vi "hdf5 image save.vi"(6 "class path":path, 7 "Save Image Path":path, 8 "error in (no error)":errorcluster, 9 "Status":T3, 10 "image #":i16=1, 11 "Refnum in":T2) -> (0 "error out":errorcluster)   [LabVIEW 2020, in "Point Grey Camera.lvclass"]
uses:
  Point Grey Camera.lvclass
  1st or last shot of scan.ctl
  <vilib>/vision/Image Controls.llb/IMAQ Image.ctl
panel:
  out "scan number":string
  in  "Python version":string="3.8"
  out "module path":path=path "C:/GEECS/Developers Version/source/Axel/openPMD-CCD/openpmd_ccd_labview.py"
  out "camera name":string
  out "Image Type 2":T1 items=["Grayscale (U8)", "Grayscale (I16)", "Grayscale (SGL)", "Complex (CSG)", "RGB (U32)", "HSL (U32)", "RGB (U64)", "Grayscale (U16)"]
  # "Error 1671 occurred at Python Node in Point Grey Camera.lvclass:hdf5 image save.vi->Point Grey Camera.lvclass:imaq save GEECS.vi->Point Grey Camera.lvclass:Save.vi->Device_control.vi\n\nPossible reason(s):\n\nLabVIEW: (Hex 0x687) There was an error in executing the specified function.\n\n\nModule Path: C:\\GEECS\\Developers Version\\source\\Device Drivers\\Point Grey Camera\\openpmd_ccd_labview.py\nFunction Name: open_write\nPython returned the following error: <class 'AssertionError'>\n[openPMD-CCD] You cannot define the same CCD name twice.\n\n\nCall Stack information:\n  File \"C:\\GEECS\\Developers Version\\source\\Device Drivers\\Point Grey Camera\\openpmd_ccd_labview.py\", line 31, in open_write\n    assert not ccd_name in scan, \"[openPMD-CCD] You cannot define the same CCD name twice.\"\n\nAssertionError: [openPMD-CCD] You cannot define the same CCD name twice."
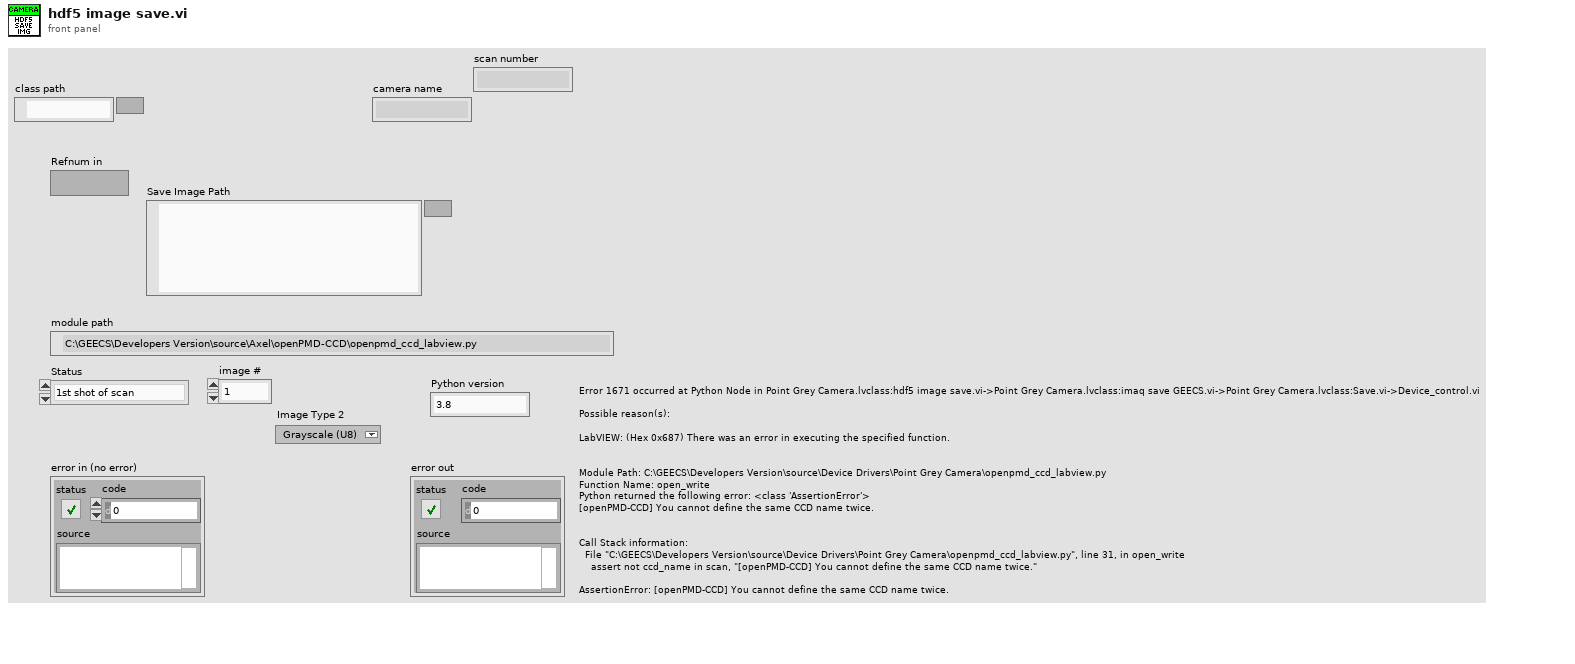
[diagram p1: front panel]
types:
  T1 = typedef "Image Type" = u32
  T2 = typedef "IMAQ Image.ctl" = refnum<image>
  T3 = typedef "1st or last shot of scan.ctl" = enum16{"1st shot of scan", "1st shot after scan end", "other"}
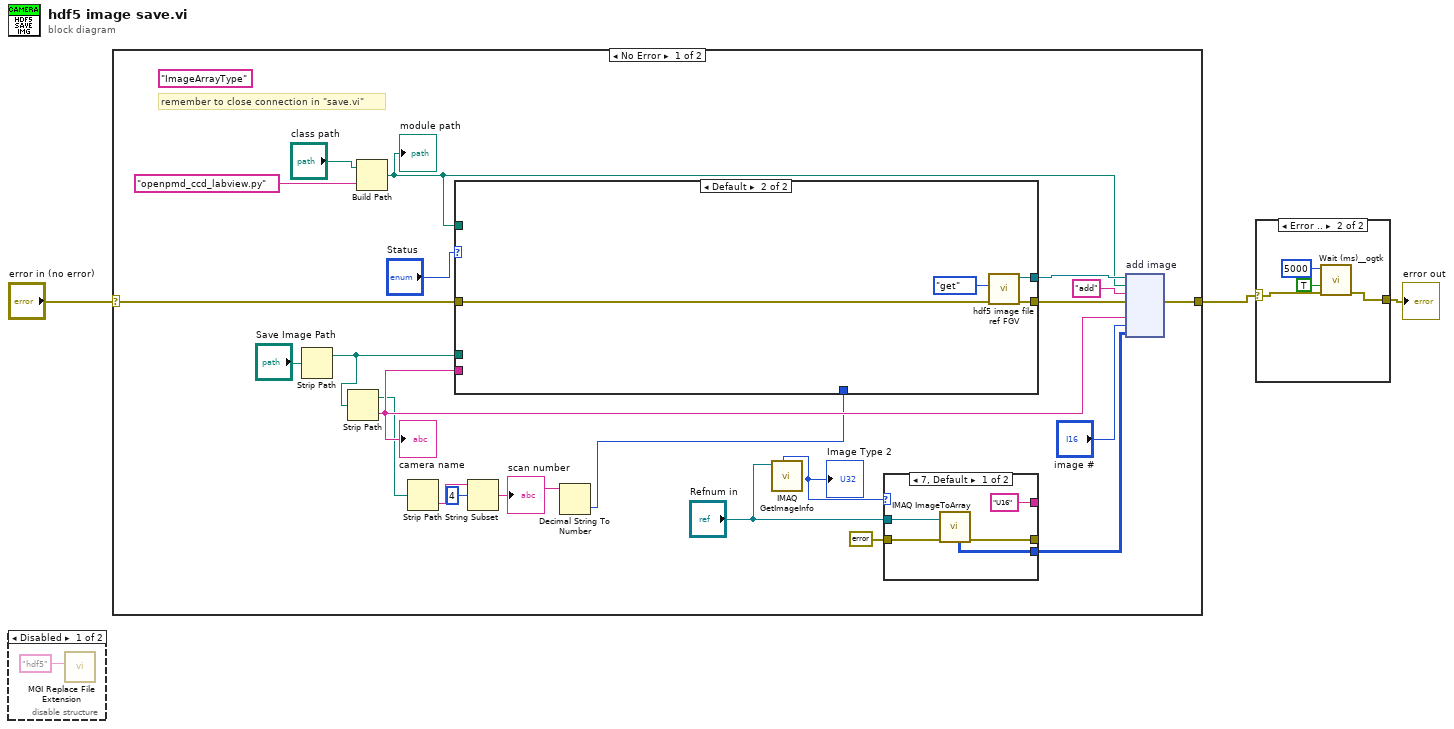
[diagram p0: block diagram]
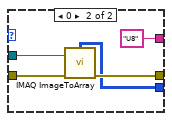
[diagram p4: hidden frame]
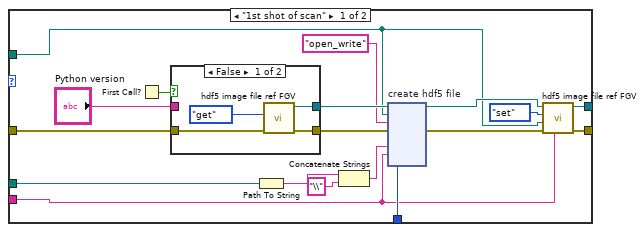
[diagram p5: hidden frame]
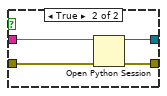
[diagram p6: hidden frame]
diagram:
  n1 = disable-structure shown="Disabled" {
    frame Disabled {
      n2 = call <userlib>:"MGI Replace File Extension.vi"("New Extension (txt)"="hdf5") -> ()  [unwired: 9 in, 2 out]
    }
    frame Enabled {
    }
  }
  n3 = case shown="No Error" "error in (no error)" {
    selector: "error in (no error)" -> [w17 w67]
    tunnel: [w19 w67] -> w2
    frame No Error {
      (unwired) "ImageArrayType"
      # "remember to close connection in \"save.vi\""
      n4 = Strip Path(path="Save Image Path") -> (stripped path=w10:path)  [unwired: 1 out]
      n5 = Strip Path(path=w10) -> (stripped path=w9:path, name=w11:string)
      "camera name" <- w11
      n6 = Build Path(base path="class path", name or relative path="openpmd_ccd_labview.py") -> (appended path=w14:path)
      "module path" <- w14
      n7 = Strip Path(path=w9) -> (name=w8:string)  [unwired: 1 out]
      n8 = String Subset(string=w8, offset (0)=4) -> (substring=w6:string)  [unwired: 1 in]
      "scan number" <- w6
      n9 = Decimal String To Number(string=w6) -> (number=w5:i32)  [unwired: 2 in, 1 out]
      n10 = case shown="Default" "Status" {
        tunnel: w17 -> [w46 w65]
        tunnel: [w41 w64] -> w15
        tunnel: w14 -> [w40 _]
        tunnel: [w44 w63] -> w18
        tunnel: w11 -> [w37 _]
        tunnel: w10 -> [w45 _]
        tunnel: w5 -> [w38 _]
        frame "1st shot of scan" {
          n11 = First Call?() -> (First Call?: T/F=w39:bool)
          n12 = case shown="False" w39 {
            tunnel: "Python version" -> [_ w62]
            tunnel: [w58 w61] -> w52
            tunnel: [w57 w60] -> w48
            tunnel: w46 -> [w55 w59]
            frame False {
              n13 = call "hdf5 image file ref FGV.vi"("error in (no error)"=w55, "command"=enum16{"set", "get"}."get") -> ("error out"=w57:errorcluster, "Python session"=w58:refnum<k35>)  [unwired: 6 in, 2 out]
            }
            frame True {
              n14 = Open Python Session(python version=w62, 3:w59) -> (session out=w61:refnum<k35>, error out=w60:errorcluster)  [unwired: 1 in]
            }
          }
          n15 = Path To String(path=w45) -> (string=w51:string)
          n16 = Concatenate Strings(w51, "\\") -> (w49:string)
          n17 = node "create hdf5 file"(w52, w40, "open_write" ("open h5 function"), w48, w49, w37, w38) -> (w43:refnum<k35>, w42:errorcluster)  [unwired: 5 in, 2 out]
          n18 = call "hdf5 image file ref FGV.vi"("Camera name"=w37, "error in (no error)"=w42, "module path in"=w40, "command"=enum16{"set", "get"}."set", "Python session"=w43) -> ("error out"=w41:errorcluster, "Python session"=w44:refnum<k35>)  [unwired: 3 in, 2 out]
        }
        frame Default {
          n19 = call "hdf5 image file ref FGV.vi"("error in (no error)"=w65, "command"=enum16{"set", "get"}."get") -> ("error out"=w64:errorcluster, "Python session"=w63:refnum<k35>)  [unwired: 6 in, 2 out]
        }
      }
      n20 = call "IMAQ GetImageInfo"("Image"="Refnum in") -> ("Image Type"=w23:T1)  [unwired: 3 in, 7 out]
      "Image Type 2" <- w23
      n21 = case shown="7, Default" w23 {
        tunnel: "Refnum in" -> [w31 w36]
        tunnel: errorcluster {"status"=FALSE, "code"=0, "source"=""} ("error in (no error)") -> [w30 w35]
        tunnel: [w29 w34] -> _
        tunnel: [w28 w33] -> w20
        tunnel: ["U16" "U8"] -> _
        frame 7, Default {
          n22 = call "IMAQ ImageToArray"("error in (no error)"=w30, "Image"=w31) -> ("Image Pixels (U16)"=w28:u16[][], "error out"=w29:errorcluster)  [unwired: 2 in, 3 out]
        }
        frame 0 {
          n23 = call "IMAQ ImageToArray"("error in (no error)"=w35, "Image"=w36) -> ("error out"=w34:errorcluster, "Image Pixels (U8)"=w33:u8[][])  [unwired: 2 in, 3 out]
        }
      }
      n24 = node "add image"(w18, w14, "add" ("function name"), w15, w11, "image #", w20) -> (w19:errorcluster)  [unwired: 5 in, 3 out]
    }
    frame Error {
    }
  }
  n25 = case shown="Error .." w2 {
    selector: w2 -> [w68 w71]
    tunnel: [w68 w72] -> w1
    frame No Error {
    }
    frame Error {
      n26 = call <userlib>:"Wait (ms)__ogtk.vi"("error in (no error)"=w71, "Wait on Error (FALSE)"=TRUE, "milliseconds to wait"=u32 5000) -> ("error out"=w72:errorcluster)  [unwired: 7 in, 1 out]
    }
  }
  "error out" <- w1
